vi "State Machine.vi"(8 "error in (no error)":errorcluster) -> (0 "error out":errorcluster)   [LabVIEW 2017, in "Toolbox.lvlib"]
uses:
  Toolbox.lvlib
  Error Handler/Error.lvlib
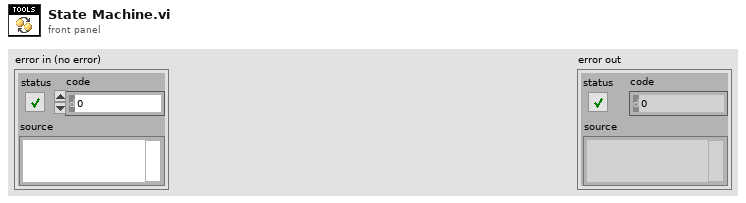
[diagram p1: front panel]
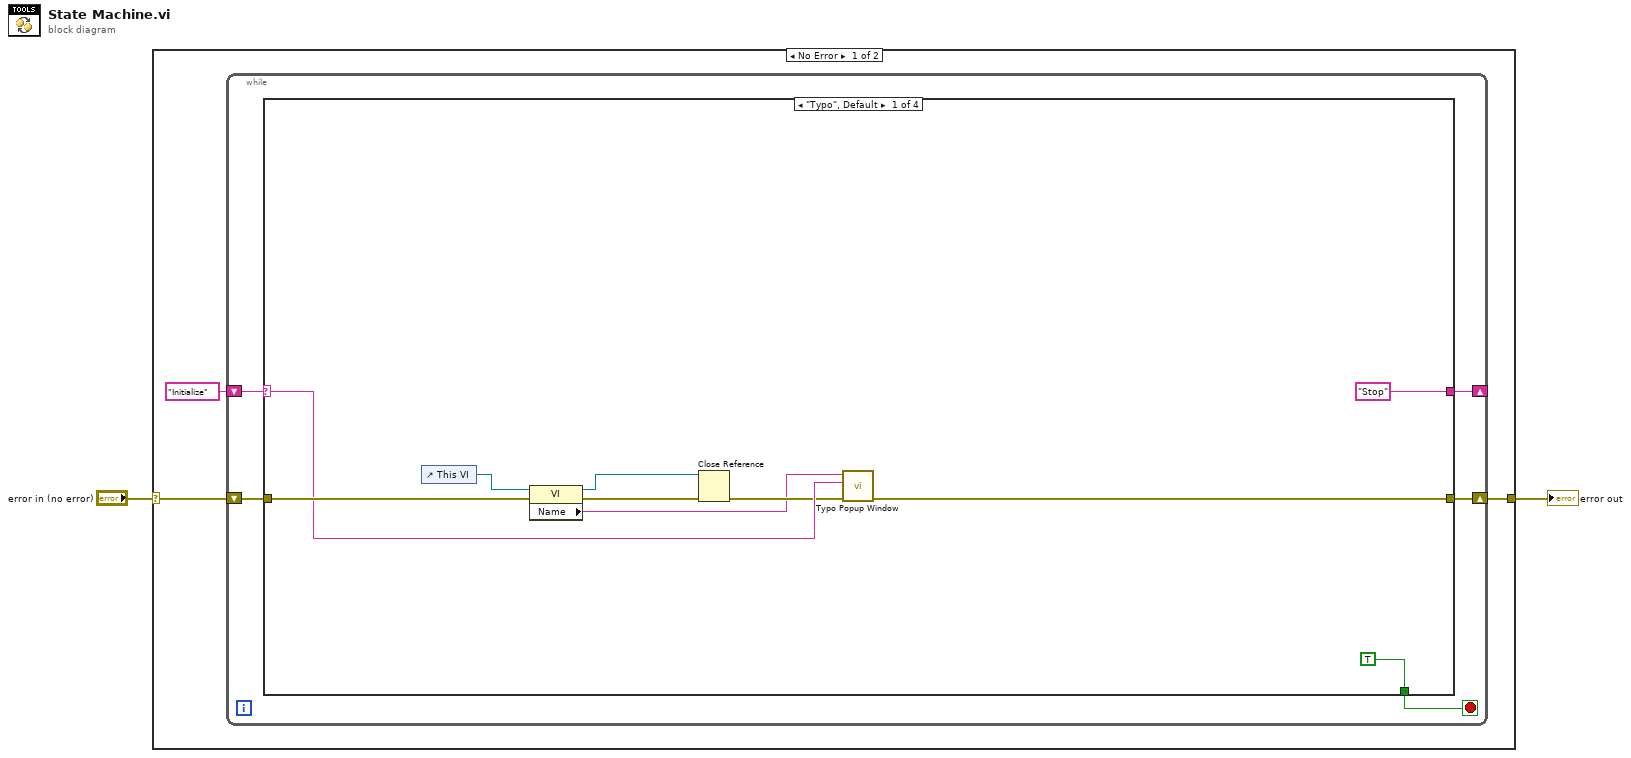
[diagram p0: block diagram]
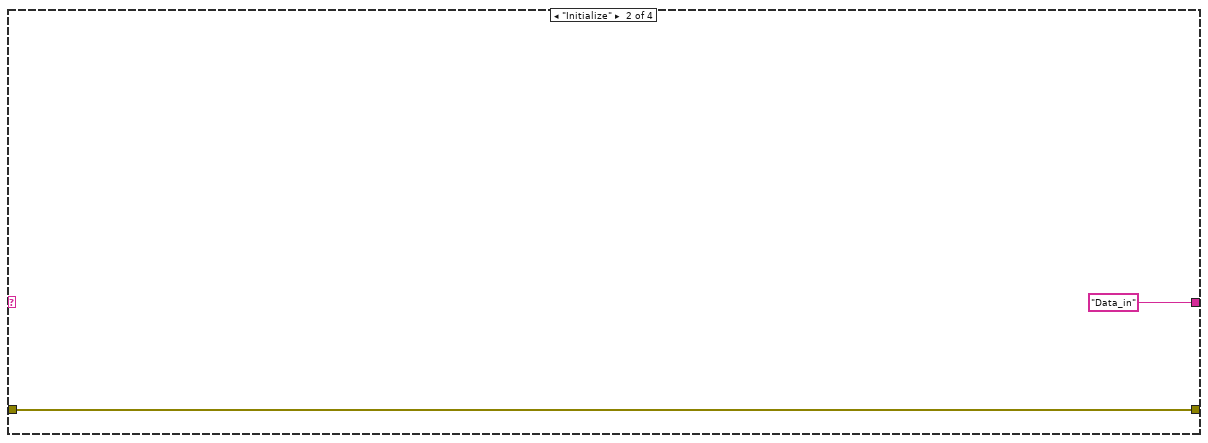
[diagram p2: hidden frame]
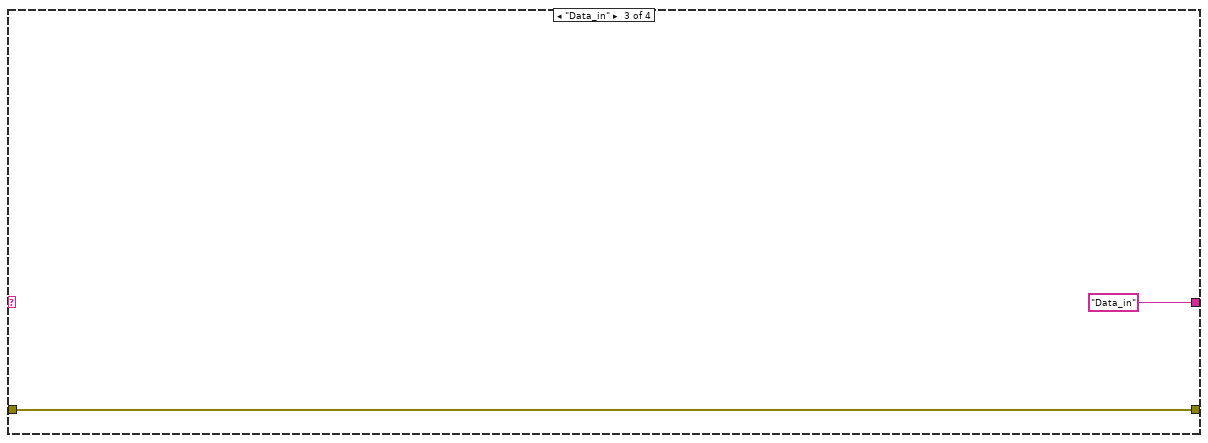
[diagram p3: hidden frame]
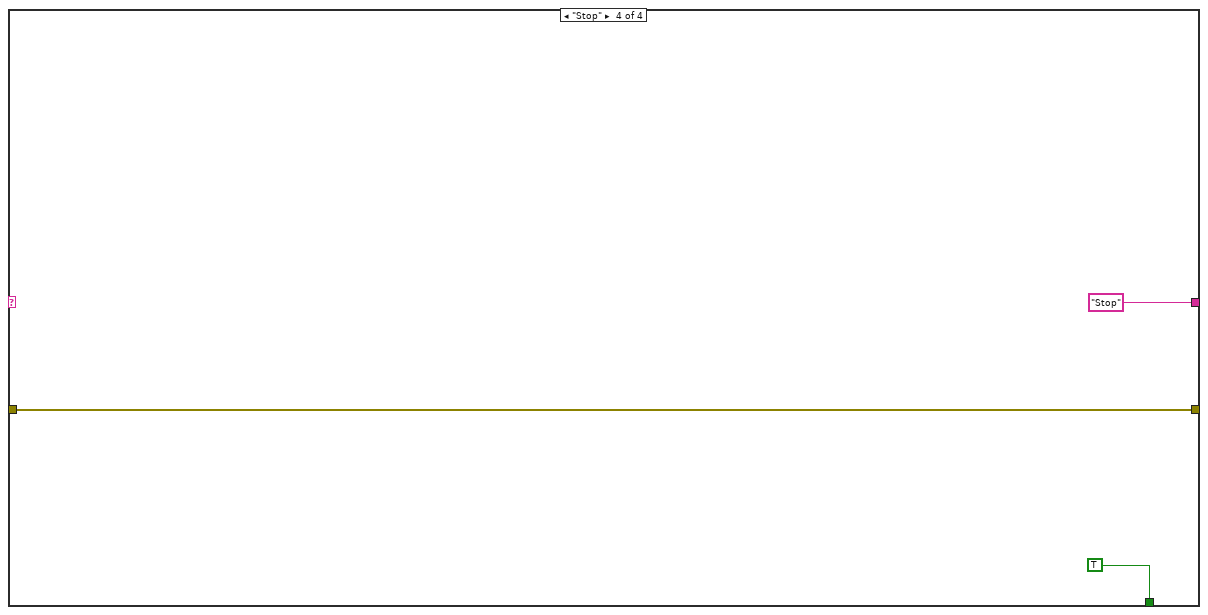
[diagram p4: hidden frame]
diagram:
  n1 = case shown="No Error" "error in (no error)" {
    selector: "error in (no error)" -> [w4 w28]
    tunnel: [w3 w28] -> w1
    frame No Error {
      n2 = while {
        shift-right: [w8] -> w3
        shift-left: w4 -> [w9]
        shift-right: [w7] -> _
        shift-left: "Initialize" -> [w10]
        stop <- w6 stop-if-true
        n3 = case shown="\"Typo\", Default" w10 {
          selector: w10 -> [w18 _ _ _]
          tunnel: w9 -> [w20 w22 w24 w27]
          tunnel: [w19 w22 w24 w27] -> w8
          tunnel: ["Stop" "Data_in" "Data_in" "Stop"] -> w7
          tunnel: [TRUE _ _ TRUE] -> w6
          frame "Typo", Default {
            n4 = control-ref of="This VI"() -> (w12:refnum<vi>)
            n5 = property class="VI"(reference=w12, error in=w20) -> (reference out=w13:refnum<vi>, error out=w15:errorcluster, "Name"=w11:string)
            n6 = Close Reference(reference=w13, error in (no error)=w15) -> (error out=w14:errorcluster)
            n7 = call "Typo Popup Window.vi"("error in (no error)"=w14, "Typo in"=w18, "VI/Loop name"=w11) -> ("error out"=w19:errorcluster)  [unwired: 8 in]
          }
          frame "Initialize" {
          }
          frame "Data_in" {
          }
          frame "Stop" {
          }
        }
      }
    }
    frame Error {
    }
  }
  "error out" <- w1
